vi "nominal_data_source.create.vi"(8 "error in":errorcluster, 9 "Description":string, 10 "ID":string, 11 "Nominal Client in":refnum<class "Nominal Client.lvclass">) -> (0 "error out":errorcluster, 1 "Created Data Source":T1, 2 "rid":string, 3 "Nominal Client out":refnum<class "Nominal Client.lvclass">)   [LabVIEW 2020, in "Nominal Client.lvclass"]
doc: "Creates a data source.\n\nid -> Required\nA human readable identifier. Must be unique within an organization. If the ID is not unique, a timestamp will be added to the ID.\n\ndescription -> Optional"
uses:
  Nominal Client.lvclass
  <vilib>/NI/Advanced HTTP Client/Header--Combo Box.ctl
  609118db-7d9c-428b-a577-7bf67d0e67c4.vi
  <vilib>/LabVIEW Open Source Project/Epoch Date & Time/formatter.iso8601/Timestamp to ISO8601 UTC DateTime.vi
  <vilib>/JDP Science/JSONtext/JSON text to Variant.vi
  <vilib>/JDP Science/JSONtext/LVClass Serializer/JSONtext LVClass Serializer.lvclass
  Nominal Client.lvclass/Nominal Client.ctl
  <vilib>/NI/Advanced HTTP Client/Session.lvclass
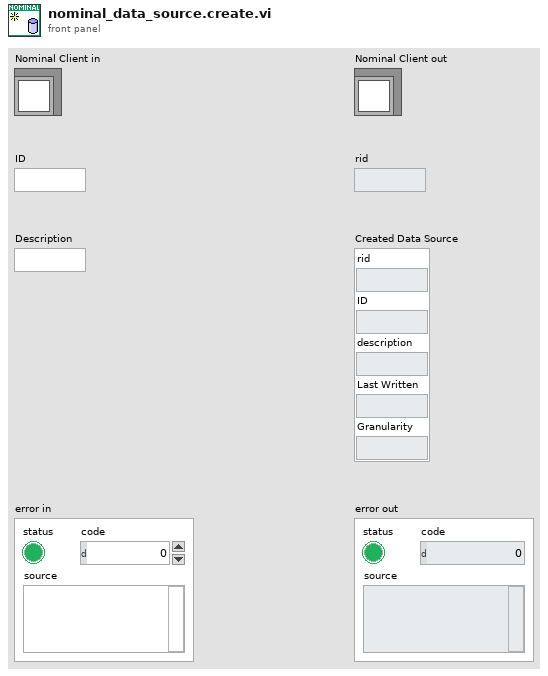
[diagram p1: front panel]
types:
  T1 = cluster{"rid":string, "ID":string, "description":string, "Last Written":string, "Granularity":string}
  T2 = typedef "lib_NI_Advanced HTTP Client.lvlib/Session.lvclass/Header--Combo Box.ctl" = string
  T3 = cluster{"rid":string, "id":string, "description":string, "dataLastWrittenAt":string, "granularity":string}
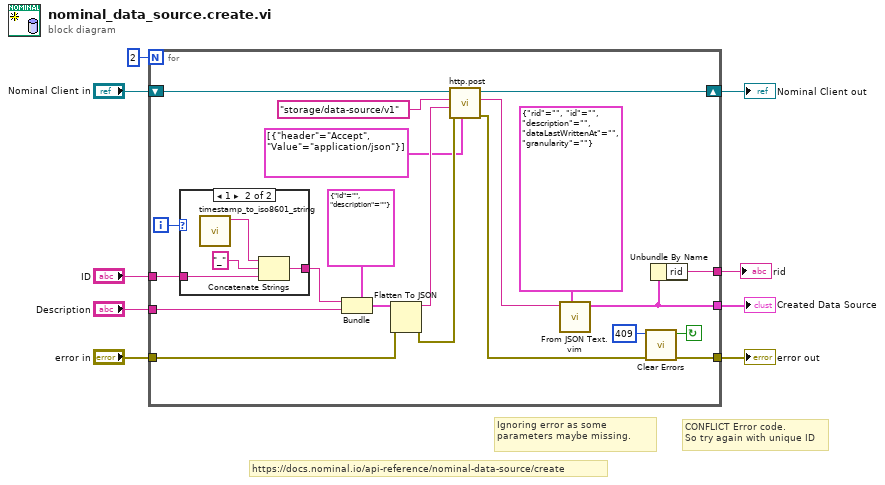
[diagram p0: block diagram]
diagram:
  # "CONFLICT Error code.\nSo try again with unique ID"
  # "Ignoring error as some parameters maybe missing."
  # "https://docs.nominal.io/api-reference/nominal-data-source/create"
  n1 = for {
    N: 2 -> [_]
    tunnel: "ID" -> [w15]
    tunnel: "Description" -> [w24]
    tunnel: [w19] -> w3
    tunnel: [w18] -> w2
    shift-right: [w29] -> w8
    shift-left: "Nominal Client in" -> [w30]
    tunnel: "error in" -> [w26]
    tunnel: [w11] -> w4
    i -> [w16]
    stop <- w10 continue-if-true
    n2 = case shown="1" w16 {
      tunnel: w15 -> [w31 w35]
      tunnel: [w31 w34] -> w14
      frame 0, Default {
      }
      frame 1 {
        n3 = call "timestamp_to_iso8601_string.vi"() -> ("ISO8601 UTC DateTime"=w32:string)  [unwired: 11 in]
        n4 = Concatenate Strings(w32, "_" ("string"), w35) -> (w34:string)
      }
    }
    n5 = Bundle(cluster=cluster{"id":string, "description":string} {"id"="", "description"=""}, "id"=w14, "description"=w24) -> (w27:cluster{"id":string, "description":string})
    n6 = Flatten To JSON(anything=w27, error in (no error)=w26) -> (JSON string=w22:string, 11:w25:errorcluster)  [unwired: 1 in]
    n7 = call "http.post.vi"("specific headers in"=cluster{"header":T2, "Value":string}[] [{"header"="Accept", "Value"="application/json"}], "error in"=w25, "Request body"=w22, "Path"="storage/data-source/v1", "Nominal Client in"=w30) -> ("error out"=w12:errorcluster, "Response"=w21:string, "Nominal Client out"=w29:refnum<class "Nominal Client.lvclass">)  [unwired: 3 in, 1 out]
    n8 = call "From JSON Text.vim"("Data Type and Default Value"=T3 {"rid"="", "id"="", "description"="", "dataLastWrittenAt"="", "granularity"=""}, "JSON"=w21) -> ("Data out"=w19:T3)  [unwired: 8 in, 1 out]
    n9 = call <vilib>:"Clear Errors.vi"("error in (no error)"=w12, "specific error code to clear (0: all)"=409) -> ("error out"=w11:errorcluster, "specific error cleared?"=w10:bool)  [unwired: 4 in]
    n10 = Unbundle By Name(w19) -> ("rid"=w18:string)
  }
  "Nominal Client out" <- w8
  "error out" <- w4
  "Created Data Source" <- w3
  "rid" <- w2
